vi "15T_Queue_Commands.vi"(1 "15T-Control":T1={"Setpoint (T)"=3.4572, "Rate (T/min)"=0.0, "Go to zero"=FALSE, "Go to Hold"=FALSE, "Go to Set"=FALSE, "Clamp"=FALSE, "Switch Heater"=FALSE} {"Rate (T/min)" format="%6_5f"; "Setpoint (T)" format="%6_5f"}, 3 "15T Queue":refnum<queue>) -> (0 "New Status":T1={"Setpoint (T)"=3.4572, "Rate (T/min)"=0.0, "Go to zero"=FALSE, "Go to Hold"=FALSE, "Go to Set"=FALSE, "Clamp"=FALSE, "Switch Heater"=FALSE} {"Rate (T/min)" format="%6_5f"; "Setpoint (T)" format="%6_5f"})   [LabVIEW 2019]
uses:
  Berta/15T-Control.ctl
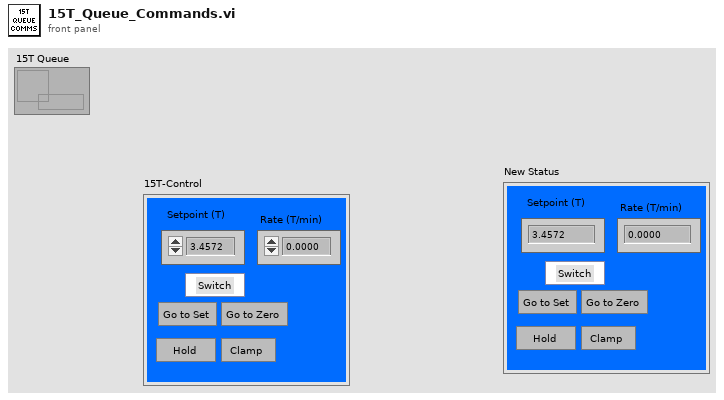
[diagram p1: front panel]
types:
  T1 = typedef "15T-Control.ctl" = cluster{"Setpoint (T)":dbl, "Rate (T/min)":dbl, "Go to zero":bool, "Go to Hold":bool, "Go to Set":bool, "Clamp":bool, "Switch Heater":bool}
  T2 = cluster{"Setpoint (T)":bool, "Rate (T/min)":bool, "Go to zero":bool, "Go to Hold":bool, "Go to Set":bool, "Clamp":bool, "Switch Heater":bool}
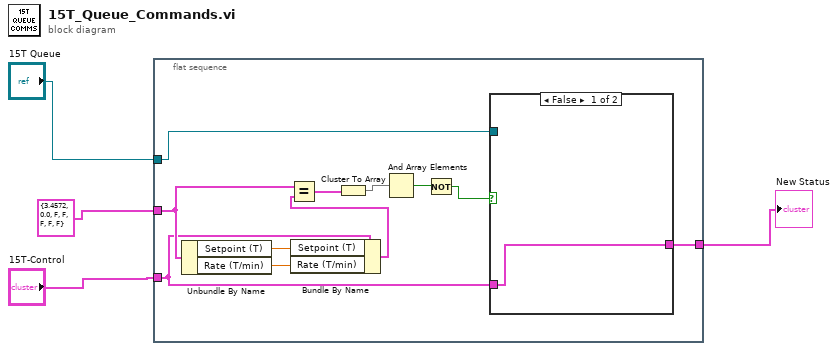
[diagram p0: block diagram]
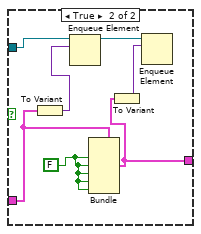
[diagram p2: hidden frame]
diagram:
  n1 = flat-sequence {
    tunnel: "15T Queue" -> [w15]
    tunnel: T1 {"Setpoint (T)"=3.4572, "Rate (T/min)"=0.0, "Go to zero"=FALSE, "Go to Hold"=FALSE, "Go to Set"=FALSE, "Clamp"=FALSE, "Switch Heater"=FALSE} ("15T-Control") -> [w11]
    tunnel: "15T-Control" -> [w10]
    tunnel: [w5] -> w1
    frame #0 {
      n2 = Unbundle By Name(w11) -> ("Setpoint (T)"=w14:dbl, "Rate (T/min)"=w13:dbl)
      n3 = Bundle By Name(cluster=w10, "Setpoint (T)"=w14, "Rate (T/min)"=w13) -> (w12:T1)
      n4 = Equal?(x=w11, y=w12) -> (x = y?=w9:T2)
      n5 = Cluster To Array(cluster=w9) -> (array=w8:bool[])
      n6 = And Array Elements(Boolean array=w8) -> (logical AND=w7:bool)
      n7 = Not(x=w7) -> (.not. x?=w6:bool)
      n8 = case shown="False" w6 {
        tunnel: w15 -> [_ w23]
        tunnel: w10 -> [w16 w21]
        tunnel: [w16 w17] -> w5
        frame False {
        }
        frame True {
          w20 = FALSE
          n9 = To Variant(anything=w21) -> (Variant=w22:variant)
          n10 = Enqueue Element(queue=w23, element=w22) -> (queue out=w19:refnum<queue>)  [unwired: 2 in, 2 out]
          n11 = Bundle(cluster=w21, "Go to zero"=w20, "Go to Hold"=w20, "Go to Set"=w20, "Clamp"=w20, "Switch Heater"=w20) -> (w17:T1)  [unwired: 2 in]
          n12 = To Variant(anything=w17) -> (Variant=w18:variant)
          n13 = Enqueue Element(queue=w19, element=w18) -> ()  [unwired: 2 in, 3 out]
        }
      }
    }
  }
  "New Status" <- w1
